vi "SetPlcSync.vi"(3 "Mode":enum16{"50Hz", "60Hz", "None"}(ring)=enum."None", 4 "Device":u8=1, 5 "Serial port":refnum<visa-resource-name>) -> (1 "Device out":u8=1, 2 "Serial port out":refnum<visa-resource-name>)   [LabVIEW 2021]
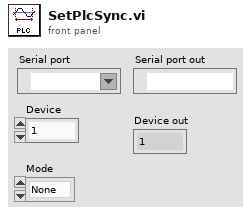
[diagram p1: front panel]
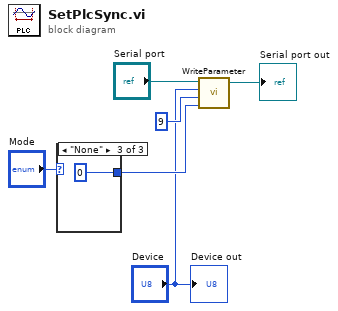
[diagram p0: block diagram]
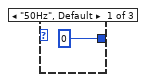
[diagram p2: hidden frame]
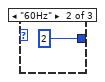
[diagram p3: hidden frame]
diagram:
  n1 = case shown="\"None\"" "Mode" {
    tunnel: [0 2 0] -> w2
    frame "50Hz", Default {
    }
    frame "60Hz" {
    }
    frame "None" {
    }
  }
  n2 = call "WriteParameter.vi"("Value"=w2, "Address"=u32 9, "Device"="Device", "Serial port"="Serial port") -> ("Serial port out"=→"Serial port out":refnum<visa-resource-name>)  [unwired: 2 in]
  "Device out" <- "Device"
